vi "ESP example 1.vi"() -> ()   [LabVIEW 2017]
panel:
  in  "Motor OFF":bool
  in  "Axis":i32=1 min=1 max=6
  in  "Target position":dbl format="%.3f"
  in  "Move":bool
  in  "Get position":bool
  in  "Motor ON":bool
  out "Position status":dbl format="%.3f"
  # "Communication is set for Com1 and default ESP controller settings.\nTo make changes, modify the appropriate parameters on the wiring diagram."
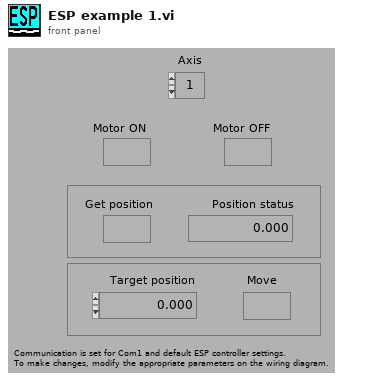
[diagram p1: front panel]
types:
  T1 = cluster{"input XON/XOFF":bool, "input HW Handshake":bool, "input alt HW HShk":bool, "output XON/XOFF":bool, "output HW Handshake":bool, "output alt HW HShk":bool, "XOFF byte":u8, "XON byte":u8, "parity error byte":u16}
  T2 = enum16{"no parity", "odd parity", "even parity", "mark parity", "space parity"}
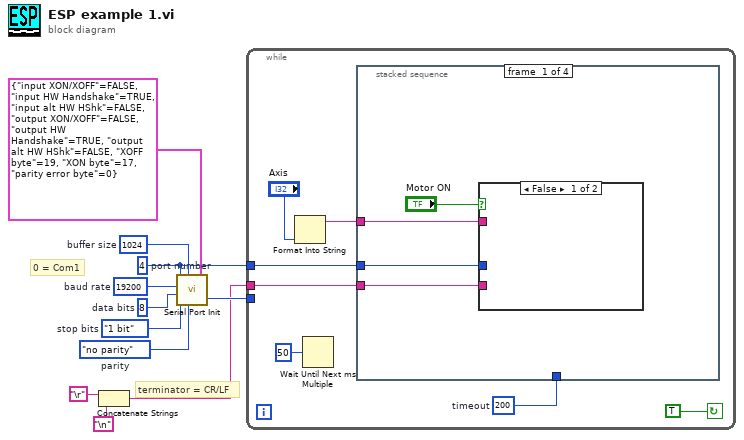
[diagram p0: block diagram]
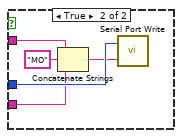
[diagram p2: hidden frame]
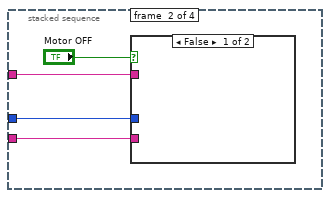
[diagram p3: hidden frame]
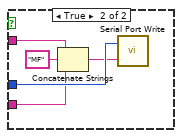
[diagram p4: hidden frame]
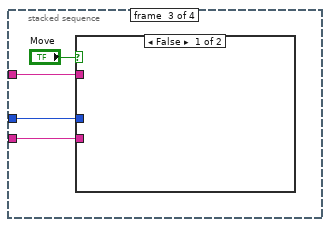
[diagram p5: hidden frame]
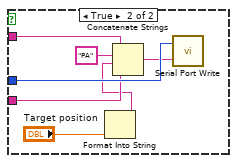
[diagram p6: hidden frame]
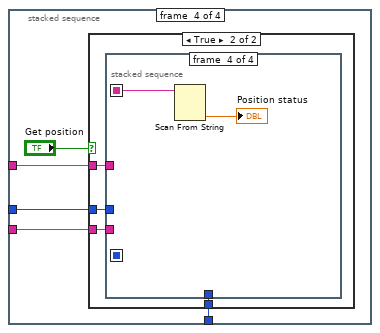
[diagram p7: hidden frame]
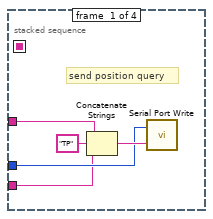
[diagram p9: hidden frame]
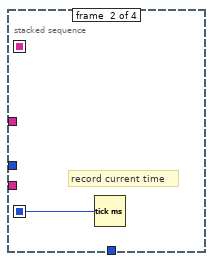
[diagram p10: hidden frame]
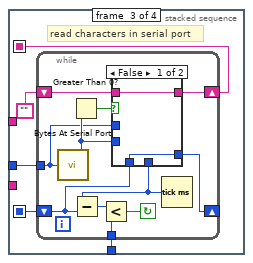
[diagram p11: hidden frame]
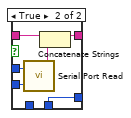
[diagram p12: hidden frame]
diagram:
  w7 = u32 19200  # baud rate
  w8 = u16 8  # data bits
  w9 = enum16{"1 bit", "1.5 bits", "2 bits"}."1 bit"  # stop bits
  w10 = T2."no parity"  # parity
  w1 = 4  # port number
  w11 = u16 1024  # buffer size
  # "terminator = CR/LF"
  # "0 = Com1"
  n1 = Concatenate Strings("\r", "\n") -> (w2:string)
  n2 = call <vilib>:"Serial Port Init.vi"("flow control etc."=T1 {"input XON/XOFF"=FALSE, "input HW Handshake"=TRUE, "input alt HW HShk"=FALSE, "output XON/XOFF"=FALSE, "output HW Handshake"=TRUE, "output alt HW HShk"=FALSE, "XOFF byte"=19, "XON byte"=17, "parity error byte"=0}, "parity"=w10, "buffer size"=w11, "stop bits"=w9, "data bits"=w8, "baud rate"=w7, "port number"=w1) -> ("error code"=w5:i32)
  n3 = while {
    tunnel: w1 -> [w13]
    tunnel: w2 -> [w14]
    tunnel: w5 -> [_]
    stop <- TRUE continue-if-true
    w12 = u32 200  # timeout
    n4 = Format Into String("Axis") -> (resulting string=w15:string)  [unwired: 3 in, 1 out]
    n5 = Wait Until Next ms Multiple(millisecond multiple=u32 50) -> ()  [unwired: 1 out]
    n6 = stacked-sequence {
      tunnel: w15 -> [w20 w30 w39 w51]
      tunnel: w14 -> [w19 w29 w38 w48]
      tunnel: w13 -> [w21 w31 w40 w50]
      tunnel: w12 -> [_ _ _ w49]
      frame #0 {
        n7 = case shown="False" "Motor ON" {
          tunnel: w21 -> [_ w27]
          tunnel: w20 -> [_ w24]
          tunnel: w19 -> [_ w23]
          frame False {
          }
          frame True {
            n8 = Concatenate Strings(w24, "MO" ("Substring"), w23) -> (w25:string)
            n9 = call <vilib>:"Serial Port Write.vi"("string to write"=w25, "port number"=w27) -> ()  [unwired: 1 out]
          }
        }
      }
      frame #1 {
        n10 = case shown="False" "Motor OFF" {
          tunnel: w31 -> [_ w36]
          tunnel: w30 -> [_ w33]
          tunnel: w29 -> [_ w32]
          frame False {
          }
          frame True {
            n11 = Concatenate Strings(w33, "MF" ("Substring"), w32) -> (w34:string)
            n12 = call <vilib>:"Serial Port Write.vi"("string to write"=w34, "port number"=w36) -> ()  [unwired: 1 out]
          }
        }
      }
      frame #2 {
        n13 = case shown="False" "Move" {
          tunnel: w40 -> [_ w47]
          tunnel: w39 -> [_ w44]
          tunnel: w38 -> [_ w43]
          frame False {
          }
          frame True {
            n14 = Format Into String("Target position") -> (resulting string=w41:string)  [unwired: 3 in, 1 out]
            n15 = Concatenate Strings(w44, "PA" ("Substring"), w41, w43) -> (w45:string)
            n16 = call <vilib>:"Serial Port Write.vi"("string to write"=w45, "port number"=w47) -> ()  [unwired: 1 out]
          }
        }
      }
      frame #3 {
        n17 = case shown="True" "Get position" {
          tunnel: w51 -> [_ w56]
          tunnel: w50 -> [_ w55]
          tunnel: w49 -> [_ w54]
          tunnel: w48 -> [_ w53]
          frame False {
          }
          frame True {
            n18 = stacked-sequence {
              seq-local: [_ w62 _ _] -> [_ _ w64 _]
              seq-local: [_ _ w63 _] -> [_ _ _ w88]
              tunnel: w56 -> [w59 _ _ _]
              tunnel: w55 -> [w58 _ w67 _]
              tunnel: w54 -> [_ _ w65 _]
              tunnel: w53 -> [w57 _ _ _]
              frame #0 {
                # "send position query"
                n19 = Concatenate Strings(w59, "TP" ("Substring"), w57) -> (w60:string)
                n20 = call <vilib>:"Serial Port Write.vi"("string to write"=w60, "port number"=w58) -> ()  [unwired: 1 out]
              }
              frame #1 {
                # "record current time"
                n21 = Tick Count (ms)() -> (millisecond timer value=w62:u32)
              }
              frame #2 {
                # "read characters in serial port"
                n22 = while {
                  shift-left: w64 -> [w68]
                  shift-right: [w69] -> _
                  tunnel: w65 -> [w72]
                  shift-left: "" -> [w75]
                  shift-right: [w74] -> w63
                  tunnel: w67 -> [w76]
                  stop <- w71 continue-if-true
                  n23 = call <vilib>:"Bytes At Serial Port.vi"("port number"=w76) -> ("byte count"=w77:u32)  [unwired: 1 out]
                  n24 = Greater Than 0?(x=w77) -> (x > 0?=w78:bool)
                  n25 = Tick Count (ms)() -> (millisecond timer value=w70:u32)
                  n26 = Subtract(x=w70, y=w68) -> (x-y=w73:u32)
                  n27 = Less?(x=w73, y=w72) -> (x < y?=w71:bool)
                  n28 = case shown="False" w78 {
                    tunnel: w77 -> [_ w86]
                    tunnel: w76 -> [_ w85]
                    tunnel: w75 -> [w80 w83]
                    tunnel: [w80 w82] -> w74
                    tunnel: [w79 w81] -> w69
                    tunnel: w70 -> [_ w81]
                    tunnel: w68 -> [w79 _]
                    frame False {
                    }
                    frame True {
                      n29 = call <vilib>:"Serial Port Read.vi"("requested byte count"=w86, "port number"=w85) -> ("string read"=w84:string)  [unwired: 1 out]
                      n30 = Concatenate Strings(w83, w84) -> (w82:string)
                    }
                  }
                }
              }
              frame #3 {
                n31 = Scan From String(input string=w88) -> (output 1=→"Position status":dbl)  [unwired: 4 in, 3 out]
              }
            }
          }
        }
      }
    }
  }
